vi "DIO Example (B).vi"() -> ()   [LabVIEW 2011]
doc: "Control the Digital Input/Output port with binary constant values (basic version)."
uses:
  C:/Program Files/Metrohm Autolab/Autolab SDK 1.10/EcoChemie.Autolab.Sdk.dll
  EcoChemie.Autolab.Sdk.dll
panel:
  out "P1 Port C read":u8
  out "IsConnected":bool
  in  "stop":bool
  out "error out":errorcluster
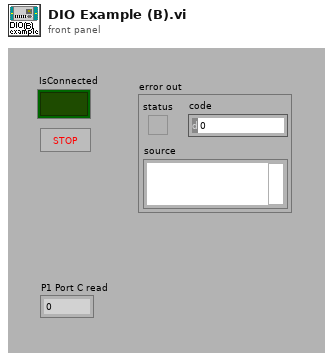
[diagram p1: front panel]
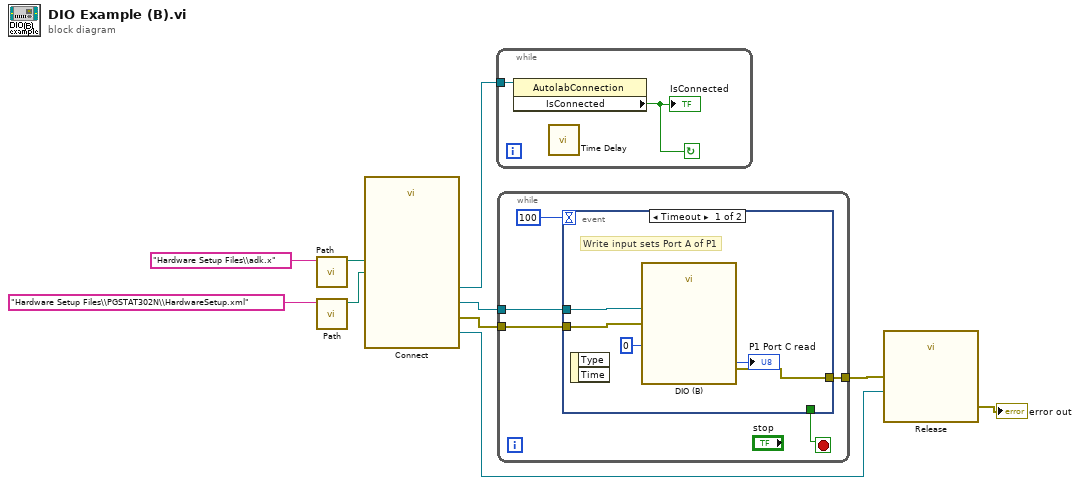
[diagram p0: block diagram]
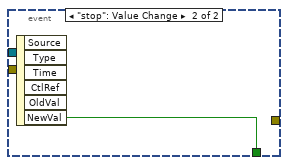
[diagram p2: hidden frame]
diagram:
  n1 = call "Path.vi"("name or relative path"="Hardware Setup Files\\adk.x") -> ("appended path"=w3:path)  [unwired: 10 in]
  n2 = call "Path.vi"("name or relative path"="Hardware Setup Files\\PGSTAT302N\\HardwareSetup.xml") -> ("appended path"=w2:path)  [unwired: 10 in]
  n3 = call "Connect.vi"("Embedded Exe File"=w3, "Hardware Setup File"=w2) -> ("Dio"=w7:refnum<k24>, "AutolabConnection"=w6:refnum<k24>, "instrument"=w9:refnum<k24>, "error out"=w8:errorcluster)  [unwired: 6 in, 4 out]
  n4 = while {
    tunnel: w6 -> [w11]
    stop <- w12 continue-if-true
    n5 = property class="AutolabConnection"(reference=w11) -> ("IsConnected"=w12:bool)  [unwired: 1 in, 2 out]
    "IsConnected" <- w12
    n6 = call "Time Delay"() -> ()  [unwired: 11 in, 1 out]
  }
  n7 = while {
    tunnel: w8 -> [w15]
    tunnel: w7 -> [w16]
    tunnel: [w13] -> w1
    stop <- w14 stop-if-true
    n8 = event shown="[0] Timeout" {
      selector: _ -> [_ _]
      dyn-events: _ -> [_ _]
      timeout: 100 ("Numeric") -> [_ _]
      tunnel: w16 -> [w20 _]
      tunnel: w15 -> [w19 _]
      tunnel: [_ w23] -> w14
      tunnel: [w18 _] -> w13
      event Timeout {
        # "Write input sets Port A of P1"
        n9 = event-data() -> ()  [unwired: 1 in, 2 out]
        n10 = call "DIO (B).vi"("error in (no error)"=w19, "Write"=u8 0 ("Value 2"), "DIO"=w20) -> ("error out"=w18:errorcluster, "Read"=→"P1 Port C read":u8)  [unwired: 7 in]
      }
      event "stop": Value Change {
        n11 = event-data() -> ("NewVal"=w23:bool)  [unwired: 1 in, 5 out]
      }
    }
  }
  n12 = call "Release.vi"("error in (no error)"=w1, "Instrument"=w9) -> ("error out"=→"error out":errorcluster)  [unwired: 9 in]
